vi "Send New Data.vi"(6 "dt":dbl, 7 "Message Priority (Normal)":T1=enum."Normal", 8 "error in (no error)":errorcluster, 9 "t0":dbl, 10 "Data":dbl[][](array[numeric]), 11 "Message Enqueuer":refnum<class "Message Enqueuer.lvclass">) -> (0 "error out":errorcluster, 3 "Message Enqueuer out":refnum<class "Message Enqueuer.lvclass">)   [LabVIEW 2020, in "VolatusData.lvlib" / "New Data Msg.lvclass"]
doc: "This VI sends the message to an actor."
uses:
  New Data Msg.lvclass
  <vilib>/ActorFramework/Message Enqueuer/Message Enqueuer.lvclass
  <vilib>/ActorFramework/Message Enqueuer/Message Priority.ctl
  C:/Program Files (x86)/National Instruments/LabVIEW 2020/vi.lib/ActorFramework/Message/Message.lvclass
  New Data Msg.lvclass/New Data Msg.ctl
  <vilib>/ActorFramework/Message Enqueuer/Message Enqueuer.lvclass/Message Enqueuer.ctl
  <vilib>/ActorFramework/Message Priority Queue/Priority Enqueue.vi
  C:/dev/lv20CE/relink/lv-volatus/Volatus/DataHandler Messages/New Data Msg/New Data Msg.lvclass
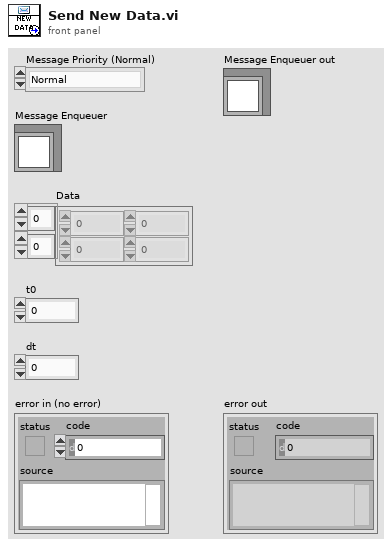
[diagram p1: front panel]
types:
  T1 = typedef "Actor Framework.lvlib/Message Enqueuer.lvclass/Message Priority.ctl" = enum16{"Low", "Normal", "High"}
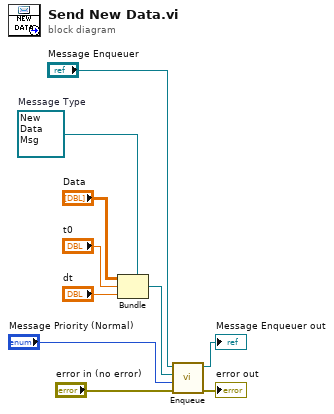
[diagram p0: block diagram]
diagram:
  w7 = refnum<class "New Data Msg.lvclass"> refnum  # Message Type
  n1 = Bundle(cluster=w7, "Data", "t0", "dt") -> (w6:refnum<class "New Data Msg.lvclass">)
  n2 = call <vilib>:"Enqueue.vi"("error in (no error)"="error in (no error)", "Message Priority (Normal)"="Message Priority (Normal)", "Message"=w6, "Message Enqueuer in"="Message Enqueuer") -> ("error out"=→"error out":errorcluster, "Message Enqueuer in"=→"Message Enqueuer out":refnum<class "Message Enqueuer.lvclass">)  [unwired: 6 in]
